vi "Is String Number.vi"(1 "String":string) -> (0 "digit?":bool)   [LabVIEW 2019]
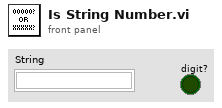
[diagram p1: front panel]
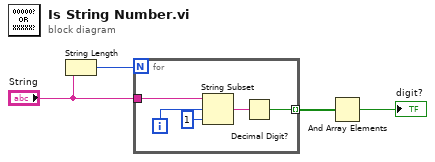
[diagram p0: block diagram]
diagram:
  n1 = String Length(string="String") -> (length=w4:i32)
  n2 = for {
    N: w4 -> [_]
    tunnel: "String" -> [w9]
    tunnel: [w6] -> w3 mode=indexing
    i -> [w7]
    n3 = String Subset(string=w9, offset (0)=w7, length (rest)=1 ("length (rest)")) -> (substring=w5:string)
    n4 = Decimal Digit?(1:w5) -> (0:w6:bool)
  }
  n5 = And Array Elements(Boolean array=w3) -> (logical AND=→"digit?":bool)
